vi "SIOSIfmDemo.vi"() -> ()   [LabVIEW 2009]
uses:
  SubVIs/Globals.vi
  <vilib>/Platform/TimedLoop/XDataNode/XDataNode.xnode
  <vilib>/Platform/TimedLoop/XDataNode/loadlvalarms.vi
  <vilib>/Platform/TimedLoop/XDataNode/timing_clust.ctl
  <vilib>/Platform/TimedLoop/XDataNode/nitl_modes.ctl
  <vilib>/Platform/TimedLoop/XDataNode/wakeup.ctl
  Instance           4 19Saved   SIOSIfmDemo .vi
  Instance           9 19Saved   SIOSIfmDemo .vi
  SIOS_IfmDLL/siosifm.dll
  <vilib>/Platform/TimedLoop/XDataNode/XDNodeRunTimeDep.lvlib
panel:
  in  "Registerkarte":T1(tab)
  out "Firmwareversion and date of compilation":string
  in  "COMNumber":i32=1 min=1 step=1
  in  "OpenCom":bool
  in  "Close":bool
  in  "CloseDevice":bool
  in  "OpenUSB":bool
  in  "Available Devices":i32(ring) items=["     1"]
  in  "SearchUSBDevices":bool
  in  "Init":bool
  in  "SetToZero":bool
  in  "StopMeasurement":bool
  in  "StartMeasurement":bool
  in  "GetMeasurement":bool
  in  "FireTrigger":bool
  in  "SetMeasurement":bool
  in  "StopSave":bool
  in  "SaveData":bool
  in  "Edge (on trigger input)":enum32{"Falling", "Rising"}(radio)
  in  "Start/Stop input":T2(radio)
  in  "Sample Clock":enum32{"Internal", "External"}(radio)
  in  "Edge (on clock input)":enum32{"Falling", "Rising"}(radio)
  in  "Hardware Trigger":bool
  in  "Edge (on event input)":enum32{"Falling", "Rising"}(radio)
  in  "Event input":enum32{"No function", "Single value"}(radio)
  in  "SampleCount":bool
  in  "Clock counter":bool
  in  "Circle":bool
  in  "SinCos":bool
  in  "Pattern":bool
  in  "Length":bool
  in  "OptionsFieldFilter":T3(radio)
  in  "Output word rate":dbl min=0.0 max=15000.0 step=10.0
  in  "Counter values":bool
  out "Channel 4":dbl
  out "Channel 3":dbl
  out "Channel 2":dbl
  out "Channel 1":dbl
  in  "Channel 4":bool
  in  "Channel 3":bool
  in  "Channel 2":bool
  in  "Channel 1":bool
  out "Estimated Outputwordrate":dbl format="%#_8f"
  in  "SetFilterBlockMode":bool
  in  "GetFilter":bool
  in  "FilterStage1NotchFreq":dbl caption="Channel 4" min=0.0
  in  "FilterStage1Ch4":dbl caption="Channel 4" min=0.0
  in  "FilterStage1Ch3":dbl caption="Channel 3" min=0.0
  in  "FilterStage1Ch2":dbl caption="Channel 2" min=0.0
  in  "FilterStage1Ch1":dbl caption="Channel 1" min=0.0
  in  "OptionFieldFilterStage1":T4(radio)
  in  "Filterstage2Val":u8 caption="2 to the power of"
  in  "9 times averaging active":bool
  in  "6 times averaging active":bool
  in  "5 times averaging active":bool
  in  "Filter stage 2":bool
  in  "Filter stage 1":bool
  in  "AVG1":u8 caption="2 to the power of"
  # "1. Initialze the DLL\n\n2. Select and open device (using USB-API or COM-port)"
  # "USB-API"
  # "COM-port"
  # "If all measurments are done, close device (Counterpart of \"OpenUSB\")"
  # "Close the library (Counterpart of \"Init\")"
  # "Signal processing options"
  # "Measurement values (length)"
  # "Measurement values selection"
  # "Filter stage 3"
  # "AVG 1"
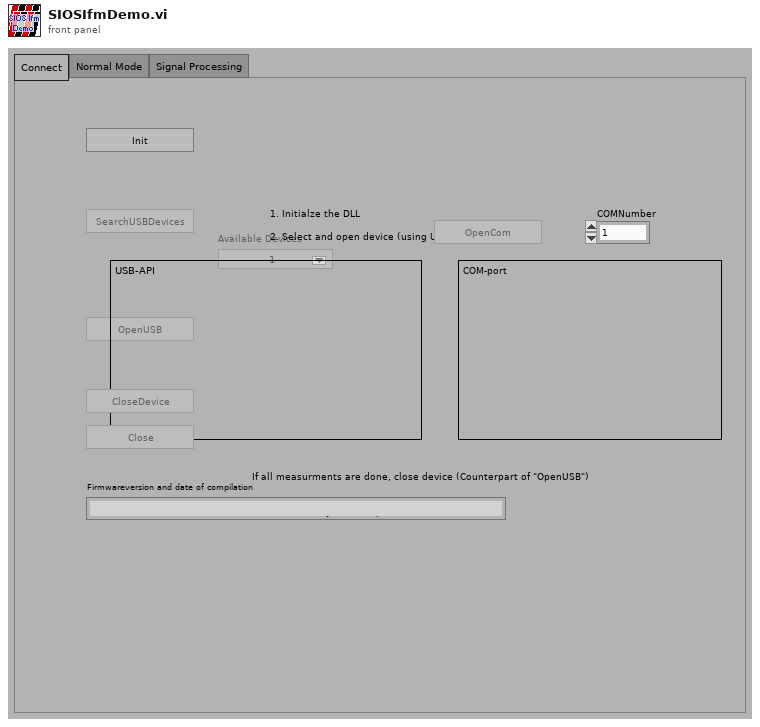
[diagram p1: front panel]
types:
  T1 = enum32{"Connect", "Normal Mode", "Signal Processing"}
  T2 = enum32{"No function", "Start trigger", "Start/Stop trigger", "Start/Stop processed"}
  T3 = enum32{"Filter off", "Filter default", "Filter user specified"}
  T4 = enum32{"FilterStage1Individual", "FilterStage1SupRefMirror", "FilterStage1NotchFilter"}
  T5 = enum8{"Enabled", "Disabled", "Disabled and Grayed Out"}
  T6 = typedef "XDNodeRunTimeDep.lvlib/timing_clust.ctl" = cluster{"Expected End [f-1]":u64, "Actual End [f-1]":u64, "Finished Late? [f-1]":bool, "Expected End [i-1]":u64, "Actual End [i-1]":u64, "Finished Late? [i-1]":bool, "Expected Start [i]":u64, "Actual Start [i]":u64, "Expected Start [f]":u64, "Actual Start [f]":u64, "Source Name":string, "Structure Name":string, "Period":i64, "Deadline":i64, "Offset":i64, "Start":i64, "Priority":i32, "Timeout":i32, "Mode":T7, "Wakeup Reason":T8, "Error":errorcluster, "Source Type":string, "Secondary Source Type":string, "Global End Time":u64, "Global Start Time":u64, "Frame Duration":u64, "Iteration Duration":u64, "Assigned CPU":i32, "I/O Scan Engine Mode":u32}
  T7 = typedef "XDNodeRunTimeDep.lvlib/nitl_modes.ctl" = enum32{"No Change", "Process missed periods, maintain original phase", "Discard missed periods, maintain original phase", "Process missed periods, ignore original phase", "Discard missed periods, ignore original phase"}
  T8 = typedef "XDNodeRunTimeDep.lvlib/wakeup.ctl" = enum32{"Normal", "Aborted", "Asynchronous wakeup", "Timing source error", "Timed loop error", "Timeout"}
  T9 = enum16{"open", "replace", "create", "open or create", "replace or create", "replace or create with confirmation"}
  T10 = cluster{"FilterOff":bool, "FilterAuto":bool, "FilterUserSpecified":bool, "FilterStage1":bool, "AVG1":i32, "FilterStage1CoeffCh1":dbl, "FilterStage1CoeffCh2":dbl, "FilterStage1CoeffCh3":dbl, "FilterStage1CoeffCh4":dbl, "FilterStage1NotchFreqCh1":dbl, "FilterStage1NotchFreqCh2":dbl, "FilterStage1NotchFreqCh3":dbl, "FilterStage1NotchFreqCh4":dbl, "FilterStage2":bool, "AVG2":i32, "5 times averaging active":bool, "6 times averaging active":bool, "9 times averaging active":bool}
  T11 = cluster{"TriggerModeOn":bool, "EventTriggerActivated":bool, "EdgeOnEventTrigger":bool, "ExternalClockActivated":bool, "EdgeOnExternalClock":bool, "TriggerStartActivated":bool, "TriggerStart/StopActivated":bool, "TriggerStart/StopProcessedActivated":bool, "EdgeOnTriggerInput":bool}
  T12 = cluster{"SendChannel1Data":bool, "SendChannel2Data":bool, "SendChannel3Data":bool, "SendChannel4Data":bool, "SendLengthValues":bool, "SendSinCosData":bool, "SendCircleData":bool, "SendTestPattern":bool, "SendClockCounterValue":bool, "SendSampleCounterValue":bool, "FilterSettings":enum32{"Auto filter", "Filter off", "Filter user specified"}, "OutputWordRate":i32}
  T13 = enum32{"Auto filter", "Filter off", "Filter user specified"}
  T14 = cluster{"Hardware Trigger":bool, "Start/Stop input":enum32{"No function", "Start trigger", "Start/Stop trigger", "Start/Stop processed"}, "Sample Clock":enum32{"Internal", "External"}, "Event input":enum32{"No function", "Single value"}, "Edge (on trigger input)":enum32{"Falling", "Rising"}, "Edge (on clock input)":enum32{"Falling", "Rising"}, "Edge (on event input)":enum32{"Falling", "Rising"}}
  T15 = cluster{"Value":bool, "Value":bool, "Value":bool, "Value":dbl, "Value":dbl, "Value":dbl, "Value":dbl, "Value":bool, "Value":dbl, "Value":bool, "Value":bool, "Value":bool, "Value":bool, "Value":u8, "Value":u8}
  T16 = cluster{"Channel 1":bool, "Channel 2":bool, "Channel 3":bool, "Channel 4":bool, "Length":bool, "SinCos":bool, "Circle":bool, "Pattern":bool, "Clock counter":bool, "SampleCount":bool, "OptionsFieldFilter":enum32{"Filter off", "Filter default", "Filter user specified"}, "Output word rate":dbl}
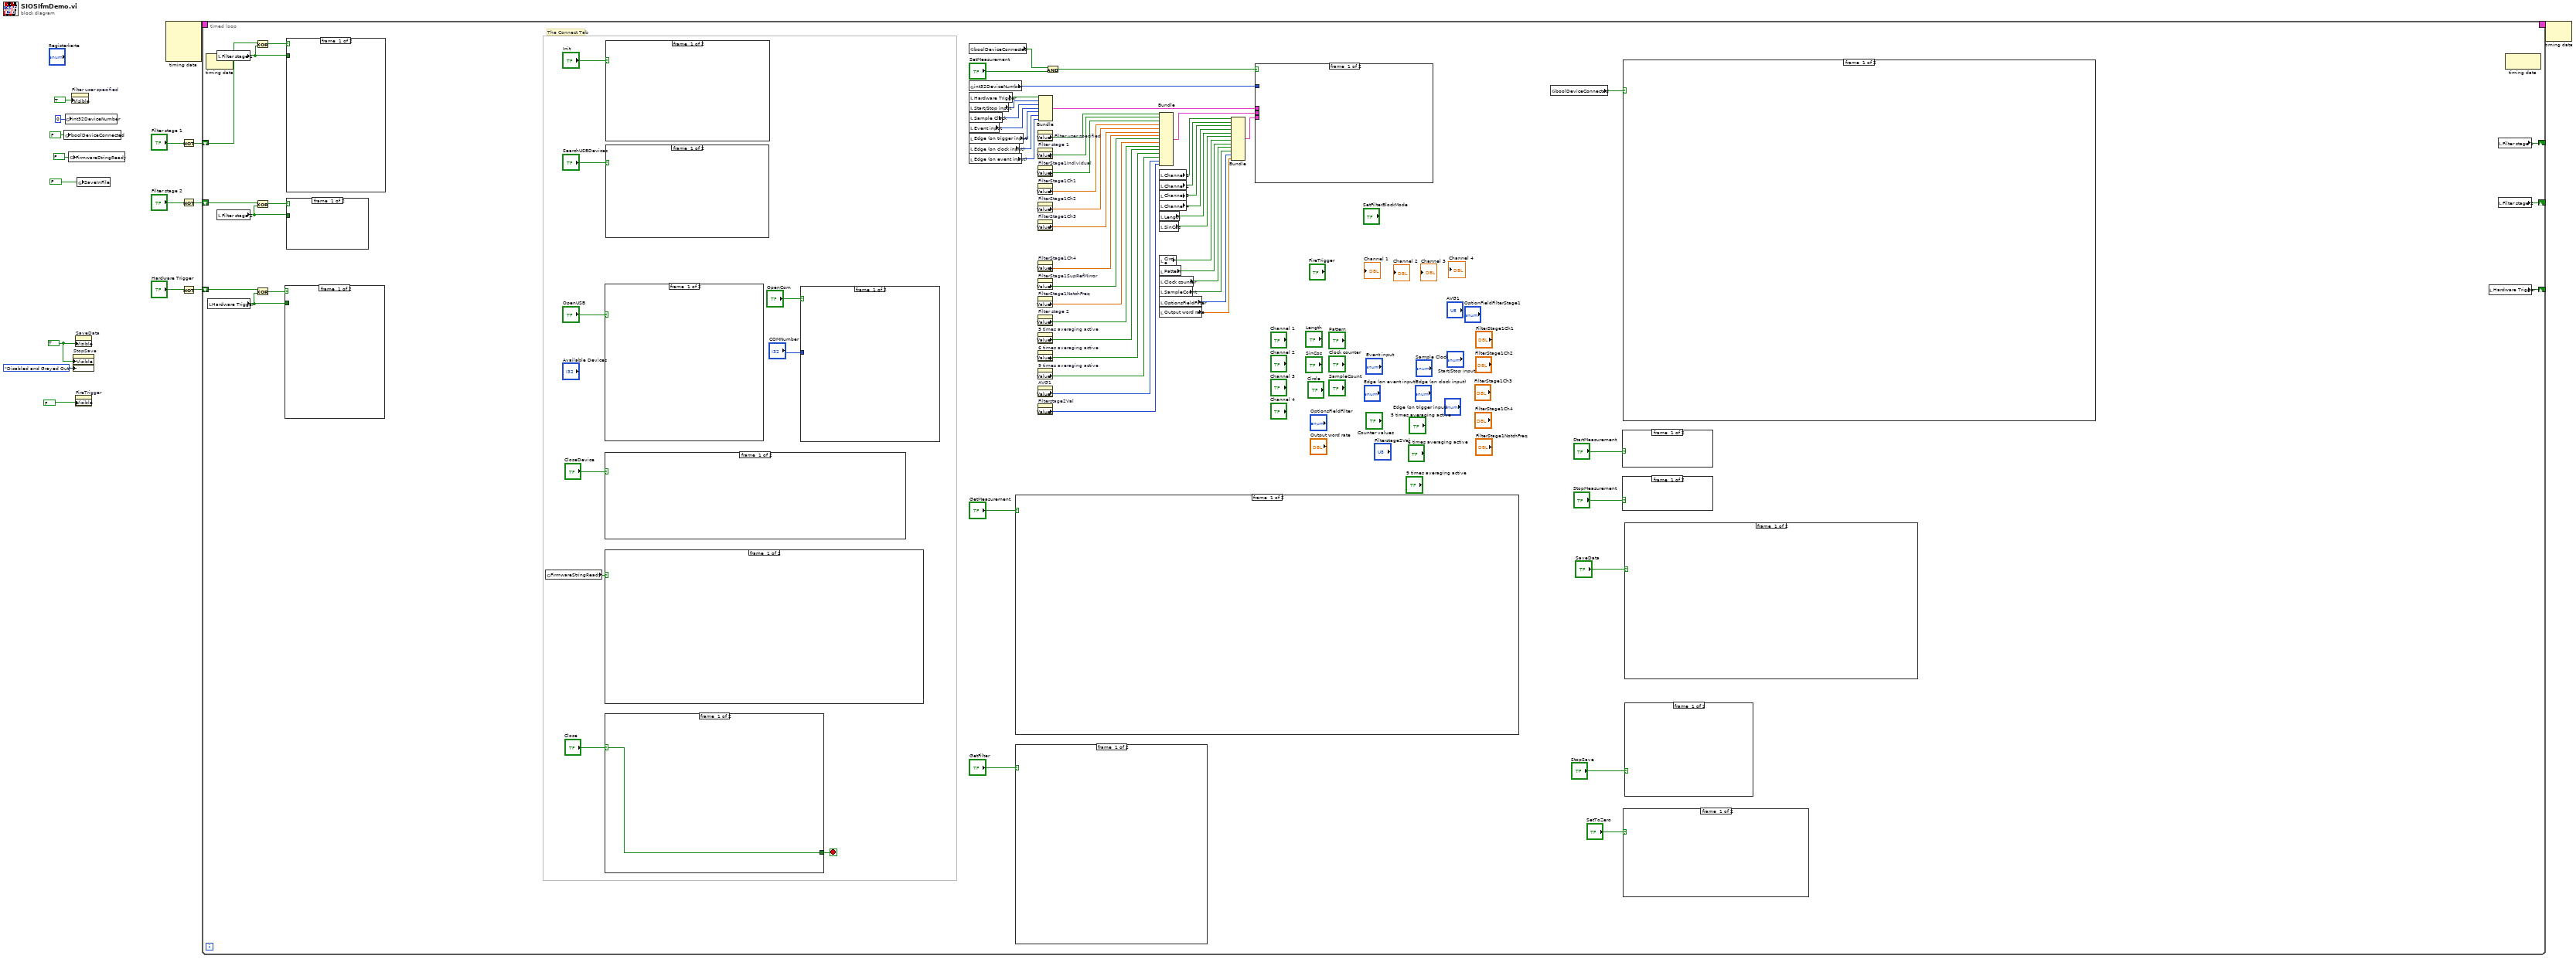
[diagram p0: block diagram]
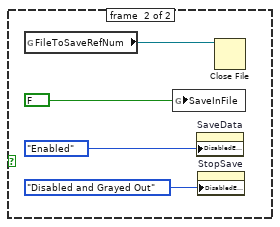
[diagram p2: hidden frame]
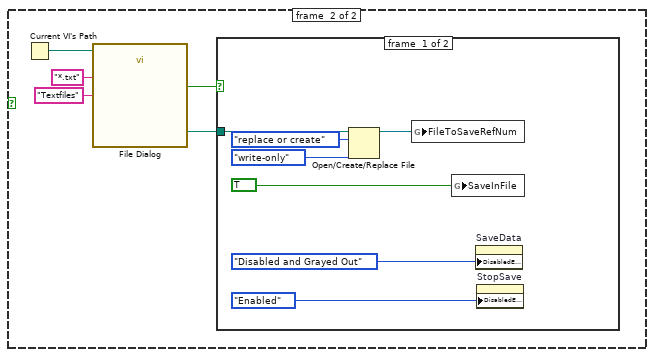
[diagram p3: hidden frame]
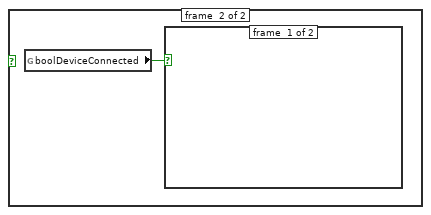
[diagram p5: hidden frame]
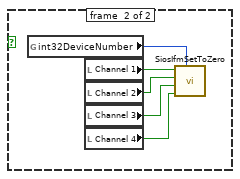
[diagram p6: hidden frame]
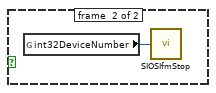
[diagram p7: hidden frame]
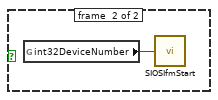
[diagram p8: hidden frame]
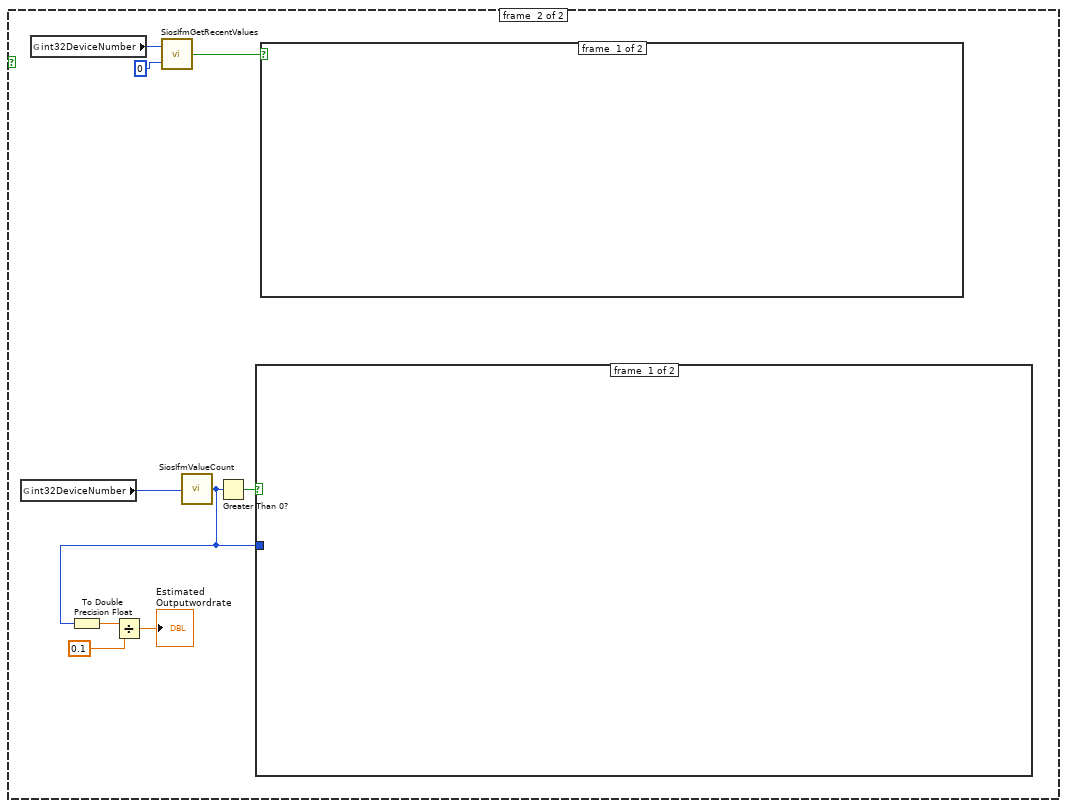
[diagram p9: hidden frame]
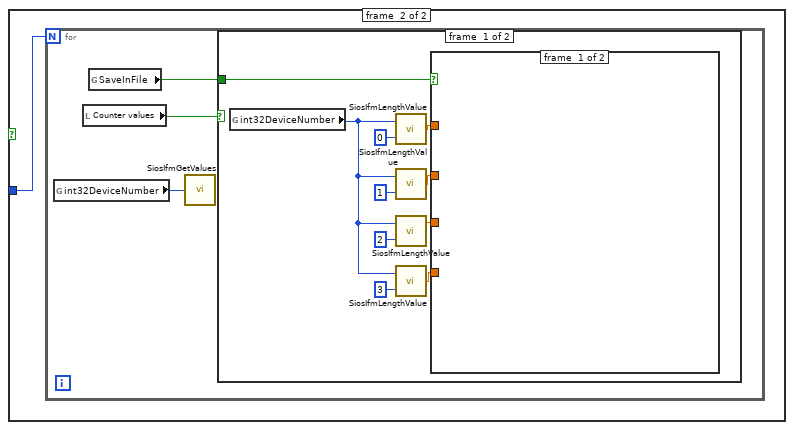
[diagram p10: hidden frame]
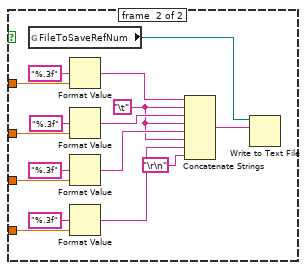
[diagram p11: hidden frame]
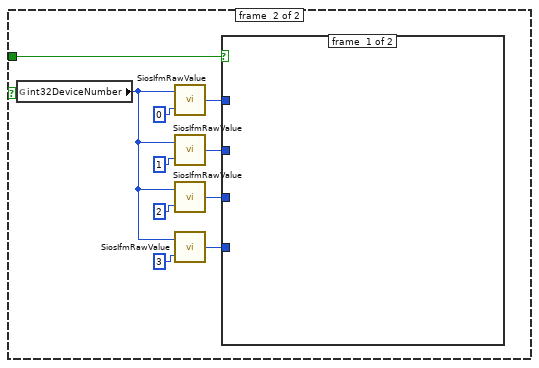
[diagram p12: hidden frame]
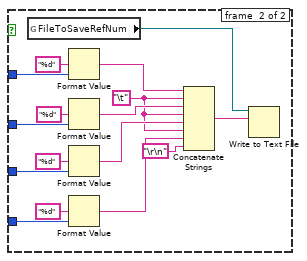
[diagram p13: hidden frame]
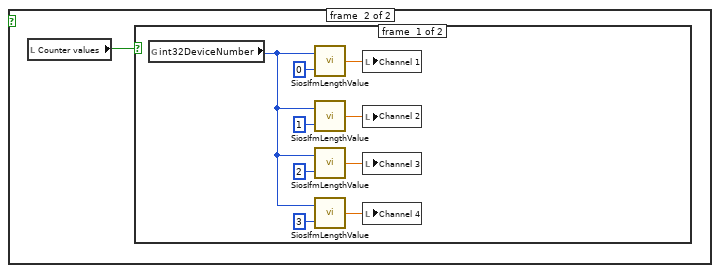
[diagram p14: hidden frame]
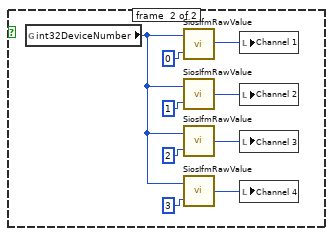
[diagram p15: hidden frame]
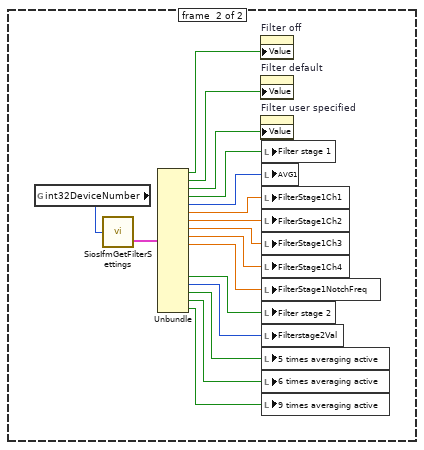
[diagram p16: hidden frame]
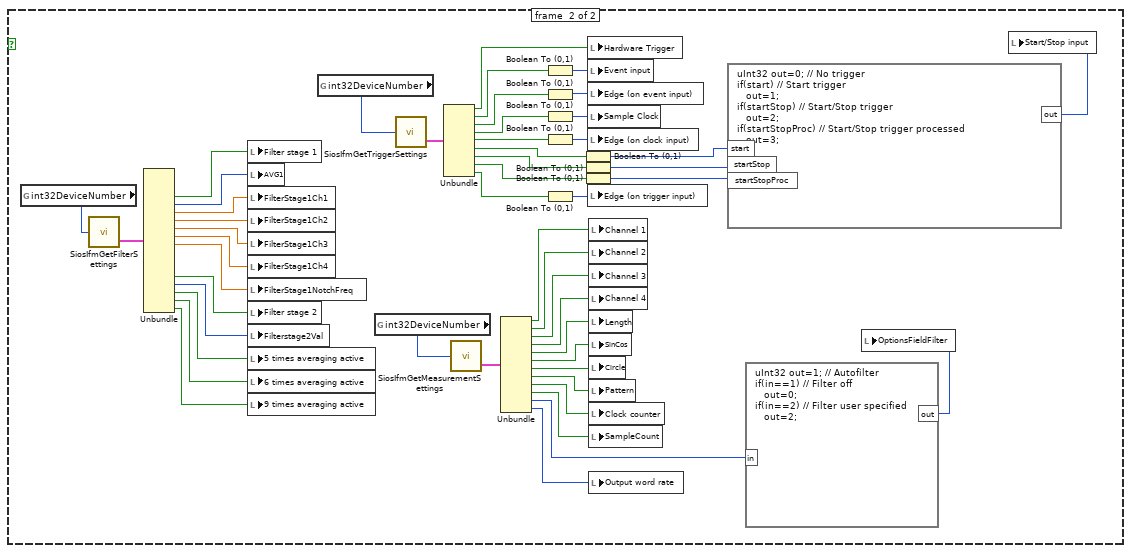
[diagram p17: hidden frame]
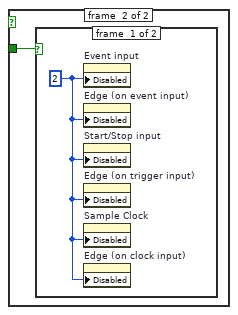
[diagram p18: hidden frame]
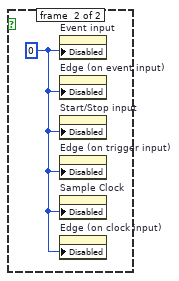
[diagram p19: hidden frame]
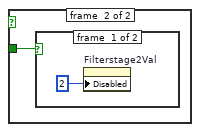
[diagram p20: hidden frame]
diagram:
  w4 = TRUE ("FirmwareStringReady")
  n1 = global write "Globals.vi" "boolDeviceConnected"(FALSE ("boolDeviceConnected")) -> ()
  n2 = global write "Globals.vi" "int32DeviceNumber"(0 ("int32DeviceNumber")) -> ()
  n3 = global write "Globals.vi" "FirmwareStringReady"(FALSE ("FirmwareStringReady")) -> ()
  n4 = property on="Filter user specified" class="Boolesch (strikt)"("Visible"=TRUE ("Sichtbar")) -> ()  [unwired: 2 in, 2 out]
  n5 = property on="StopSave" class="Bool"("Visible"=w4, "DisabledEnum"=T5."Disabled and Grayed Out" ("Disabled")) -> ()  [unwired: 2 in, 2 out]
  n6 = property on="SaveData" class="Bool"("Visible"=w4) -> ()  [unwired: 2 in, 2 out]
  n7 = property on="FireTrigger" class="Bool"("Visible"=FALSE ("FirmwareStringReady")) -> ()  [unwired: 2 in, 2 out]
  n8 = global write "Globals.vi" "SaveInFile"(FALSE ("FirmwareStringReady")) -> ()
  n9 = node-c288() -> (w6:T6)  [unwired: 4 in]
  n10 = Not(x="Filter stage 1") -> (.not. x?=w12:bool)
  n11 = Not(x="Filter stage 2") -> (.not. x?=w10:bool)
  n12 = Not(x="Hardware Trigger") -> (.not. x?=w9:bool)
  n13 = timed-loop {
    shift-right: [w55] -> _
    shift-left: w12 -> [w51]
    shift-right: [w54] -> _
    shift-left: w10 -> [w50]
    shift-right: [w52] -> _
    shift-left: w9 -> [w49]
    timing: w6 -> [_]
    timing-out: [_] -> w5
    stop <- w84 stop-if-true
    # "The Connect Tab"
    n14 = node-c288() -> ()  [unwired: 1 in, 1 out]
    n15 = local read "Hardware Trigger"() -> (w43:bool)
    n16 = local read "Filter stage 1"() -> (w47:bool)
    n17 = local read "Filter stage 2"() -> (w45:bool)
    n18 = Exclusive Or(1:w47, 2:w51) -> (0:w48:bool)
    n19 = Exclusive Or(1:w45, 2:w50) -> (0:w46:bool)
    n20 = Exclusive Or(1:w43, 2:w49) -> (0:w44:bool)
    n21 = case shown="True" w44 {
      tunnel: w43 -> [_ w263]
      frame #0 {
      }
      frame #1 {
        n22 = case shown="False" w263 {
          frame #0 {
            w264 = u8 2 ("Nicht aktiv")
            n23 = property on="Event input" class="OptionsfelderElement (strikt)"("Disabled"=w264) -> ()  [unwired: 2 in, 2 out]
            n24 = property on="Edge (on event input)" class="OptionsfelderElement (strikt)"("Disabled"=w264) -> ()  [unwired: 2 in, 2 out]
            n25 = property on="Start/Stop input" class="OptionsfelderElement (strikt)"("Disabled"=w264) -> ()  [unwired: 2 in, 2 out]
            n26 = property on="Edge (on trigger input)" class="OptionsfelderElement (strikt)"("Disabled"=w264) -> ()  [unwired: 2 in, 2 out]
            n27 = property on="Sample Clock" class="OptionsfelderElement (strikt)"("Disabled"=w264) -> ()  [unwired: 2 in, 2 out]
            n28 = property on="Edge (on clock input)" class="OptionsfelderElement (strikt)"("Disabled"=w264) -> ()  [unwired: 2 in, 2 out]
          }
          frame #1 {
            w265 = u8 0 ("Nicht aktiv")
            n29 = property on="Event input" class="OptionsfelderElement (strikt)"("Disabled"=w265) -> ()  [unwired: 2 in, 2 out]
            n30 = property on="Edge (on event input)" class="OptionsfelderElement (strikt)"("Disabled"=w265) -> ()  [unwired: 2 in, 2 out]
            n31 = property on="Start/Stop input" class="OptionsfelderElement (strikt)"("Disabled"=w265) -> ()  [unwired: 2 in, 2 out]
            n32 = property on="Edge (on trigger input)" class="OptionsfelderElement (strikt)"("Disabled"=w265) -> ()  [unwired: 2 in, 2 out]
            n33 = property on="Sample Clock" class="OptionsfelderElement (strikt)"("Disabled"=w265) -> ()  [unwired: 2 in, 2 out]
            n34 = property on="Edge (on clock input)" class="OptionsfelderElement (strikt)"("Disabled"=w265) -> ()  [unwired: 2 in, 2 out]
          }
        }
      }
    }
    n35 = case shown="True" w48 {
      tunnel: w47 -> [_ w269]
      frame #0 {
      }
      frame #1 {
        n36 = case shown="True" w269 {
          frame #0 {
            w270 = u8 2 ("Nicht aktiv")
            n37 = property on="AVG1" class="Digital (strikt)"("Disabled"=w270) -> ()  [unwired: 2 in, 2 out]
            n38 = property on="OptionFieldFilterStage1" class="OptionsfelderElement (strikt)"("Disabled"=w270) -> ()  [unwired: 2 in, 2 out]
            n39 = property on="FilterStage1Ch1" class="Digital (strikt)"("Disabled"=w270) -> ()  [unwired: 2 in, 2 out]
            n40 = property on="FilterStage1Ch2" class="DigitalWert (strikt)"("Disabled"=w270) -> ()  [unwired: 2 in, 2 out]
            n41 = property on="FilterStage1Ch3" class="DigitalWert (strikt)"("Disabled"=w270) -> ()  [unwired: 2 in, 2 out]
            n42 = property on="FilterStage1Ch4" class="DigitalWert (strikt)"("Disabled"=w270) -> ()  [unwired: 2 in, 2 out]
            n43 = property on="FilterStage1NotchFreq" class="Digital (strikt)"("Disabled"=w270) -> ()  [unwired: 2 in, 2 out]
          }
          frame #1 {
            w271 = u8 0 ("Nicht aktiv")
            n44 = property on="AVG1" class="Digital (strikt)"("Disabled"=w271) -> ()  [unwired: 2 in, 2 out]
            n45 = property on="OptionFieldFilterStage1" class="OptionsfelderElement (strikt)"("Disabled"=w271) -> ()  [unwired: 2 in, 2 out]
            n46 = property on="FilterStage1Ch1" class="Digital (strikt)"("Disabled"=w271) -> ()  [unwired: 2 in, 2 out]
            n47 = property on="FilterStage1Ch2" class="DigitalWert (strikt)"("Disabled"=w271) -> ()  [unwired: 2 in, 2 out]
            n48 = property on="FilterStage1Ch3" class="DigitalWert (strikt)"("Disabled"=w271) -> ()  [unwired: 2 in, 2 out]
            n49 = property on="FilterStage1Ch4" class="DigitalWert (strikt)"("Disabled"=w271) -> ()  [unwired: 2 in, 2 out]
            n50 = property on="FilterStage1NotchFreq" class="Digital (strikt)"("Disabled"=w271) -> ()  [unwired: 2 in, 2 out]
          }
        }
      }
    }
    n51 = case shown="True" w46 {
      tunnel: w45 -> [_ w266]
      frame #0 {
      }
      frame #1 {
        n52 = case shown="False" w266 {
          frame #0 {
            n53 = property on="Filterstage2Val" class="Digital (strikt)"("Disabled"=u8 2 ("Nicht aktiv")) -> ()  [unwired: 2 in, 2 out]
          }
          frame #1 {
            n54 = property on="Filterstage2Val" class="Digital (strikt)"("Disabled"=u8 0 ("Nicht aktiv")) -> ()  [unwired: 2 in, 2 out]
          }
        }
      }
    }
    n55 = global read "Globals.vi" "FirmwareStringReady"() -> (w78:bool)
    n56 = case shown="True" "OpenUSB" {
      frame #0 {
      }
      frame #1 {
        n57 = property on="Available Devices" class="Ring (strikt)"() -> ("Value"=w295:i32)  [unwired: 2 in, 2 out]
        n58 = call "SiosIfmOpenUSB.vi"("uniqueId"=w295) -> ("IfmOpenUSB"=w296:i32)
        n59 = Greater Or Equal To 0?(x=w296) -> (x >= 0?=w297:bool)
        n60 = case shown="True" w297 {
          tunnel: w296 -> [_ w299]
          frame #0 {
          }
          frame #1 {
            w301 = u8 2 ("Nicht aktiv")
            n61 = global write "Globals.vi" "int32DeviceNumber"(w299) -> ()
            n62 = global write "Globals.vi" "boolDeviceConnected"(TRUE ("boolDeviceConnected")) -> ()
            n63 = global write "Globals.vi" "FirmwareStringReady"(TRUE ("FirmwareStringReady")) -> ()
            n64 = property on="CloseDevice" class="Boolesch"("Disabled"=u8 0 ("Nicht aktiv")) -> ()  [unwired: 2 in, 2 out]
            n65 = property on="OpenUSB" class="Boolesch"("Disabled"=w301) -> ()  [unwired: 2 in, 2 out]
            n66 = property on="OpenCom" class="Boolesch"("Disabled"=w301) -> ()  [unwired: 2 in, 2 out]
          }
        }
      }
    }
    n67 = case shown="True" "CloseDevice" {
      frame #0 {
      }
      frame #1 {
        n68 = flat-sequence {
          frame #0 {
            n69 = global read "Globals.vi" "int32DeviceNumber"() -> (w292:i32)
            n70 = call "SiosIfmCloseDevice.vi"("DeviceNumber"=w292) -> ()
          }
          frame #1 {
            w294 = u8 0 ("Nicht aktiv")
            n71 = property on="CloseDevice" class="Boolesch"("Disabled"=u8 2 ("Nicht aktiv")) -> ()  [unwired: 2 in, 2 out]
            n72 = property on="OpenUSB" class="Boolesch"("Disabled"=w294) -> ()  [unwired: 2 in, 2 out]
            n73 = property on="OpenCom" class="Boolesch"("Disabled"=w294) -> ()  [unwired: 2 in, 2 out]
          }
        }
        n74 = global write "Globals.vi" "boolDeviceConnected"(FALSE ("boolDeviceConnected")) -> ()
      }
    }
    n75 = case shown="True" w78 {
      frame #0 {
      }
      frame #1 {
        n76 = flat-sequence {
          frame #0 {
            n77 = while {
              i -> [w285]
              stop <- w283 continue-if-true
              # "Wait until\ndevice info\nis available\nor timeout \nafter \n5 seconds."
              n78 = global read "Globals.vi" "int32DeviceNumber"() -> (w278:i32)
              n79 = Greater Or Equal?(x=50, y=w285) -> (x >= y?=w281:bool)
              n80 = call "Verzögerung"("Delay Time (s)"=0.1) -> ()  [unwired: 10 in, 1 out]
              n81 = dll-call lib="D:/Support/Labview/RE-10/SIOS_IfmDLL/siosifm.dll" fn="IfmDeviceInfo"("deviceNumber"=w278, "requestedInfo"=8) -> (w279:i32)  [unwired: 5 in, 2 out]
              n82 = Not Equal?(x=1, y=w279) -> (x != y?=w282:bool)
              n83 = And(x=w282, y=w281) -> (x .and. y?=w283:bool)
            }
          }
          frame #1 {
            n84 = global read "Globals.vi" "int32DeviceNumber"() -> (w288:i32)
            n85 = global write "Globals.vi" "FirmwareStringReady"(FALSE ("FirmwareStringReady")) -> ()
            n86 = call "SiosIfmIGetFirmwareVersion.vi"("devNumber"=w288) -> ("Ausgabe-Parameter"=→"Firmwareversion and date of compilation":string)
          }
        }
      }
    }
    n87 = case shown="True" "Close" {
      selector: "Close" -> [w317 w320]
      tunnel: [w317 w318] -> w84
      frame #0 {
      }
      frame #1 {
        n88 = flat-sequence {
          tunnel: w320 -> [w321]
          tunnel: [w321] -> w319
          tunnel: [w324] -> w318
          tunnel: w319 -> [w324]
          frame #0 {
            n89 = call "SIOSIfmClose.vi"() -> ()  [unwired: 1 in]
          }
          frame #1 {
            w323 = u8 2 ("Nicht aktiv")
            n90 = property on="Init" class="Boolesch"("Disabled"=u8 0 ("Nicht aktiv")) -> ()  [unwired: 2 in, 2 out]
            n91 = property on="SearchUSBDevices" class="Boolesch"("Disabled"=w323) -> ()  [unwired: 2 in, 2 out]
            n92 = property on="OpenUSB" class="Boolesch"("Disabled"=w323) -> ()  [unwired: 2 in, 2 out]
            n93 = property on="Available Devices" class="Ring (strikt)"("Disabled"=w323) -> ()  [unwired: 2 in, 2 out]
            n94 = global write "Globals.vi" "boolDeviceConnected"(FALSE ("boolDeviceConnected")) -> ()
            n95 = property on="CloseDevice" class="Boolesch"("Disabled"=w323) -> ()  [unwired: 2 in, 2 out]
            n96 = property on="Close" class="Boolesch"("Disabled"=w323) -> ()  [unwired: 2 in, 2 out]
            n97 = property on="OpenCom" class="Boolesch"("Disabled"=w323) -> ()  [unwired: 2 in, 2 out]
          }
        }
      }
    }
    n98 = case shown="True" "Init" {
      frame #0 {
      }
      frame #1 {
        n99 = call "SiosIfmInit.vi"() -> ("IfmInit"=w326:i32)
        n100 = Equal To 0?(x=w326) -> (x = 0?=w327:bool)
        n101 = case shown="True" w327 {
          frame #0 {
          }
          frame #1 {
            w328 = u8 0 ("Nicht aktiv")
            n102 = property on="Init" class="Boolesch"("Disabled"=u8 2 ("Nicht aktiv")) -> ()  [unwired: 2 in, 2 out]
            n103 = property on="SearchUSBDevices" class="Boolesch"("Disabled"=w328) -> ()  [unwired: 2 in, 2 out]
            n104 = property on="Close" class="Boolesch"("Disabled"=w328) -> ()  [unwired: 2 in, 2 out]
            n105 = property on="OpenCom" class="Boolesch"("Disabled"=w328) -> ()  [unwired: 2 in, 2 out]
          }
        }
      }
    }
    n106 = case shown="True" "SearchUSBDevices" {
      frame #0 {
      }
      frame #1 {
        n107 = call "SiosIfmSearchUSBDevices.vi"() -> ("Array"=w312:cluster{string, i16}[], "Number of SIOS USB Devices"=w313:i32)
        n108 = Greater Than 0?(x=w313) -> (x > 0?=w311:bool)
        n109 = case shown="True" w311 {
          tunnel: w312 -> [_ w314]
          frame #0 {
          }
          frame #1 {
            n110 = property on="Available Devices" class="Ring (strikt)"("Strings And Values []"=w314) -> ()  [unwired: 2 in, 2 out]
            n111 = property on="OpenUSB" class="Boolesch"("Disabled"=u8 0 ("Nicht aktiv")) -> ()  [unwired: 2 in, 2 out]
            n112 = property on="Available Devices" class="Ring (strikt)"("Disabled"=u8 0 ("Nicht aktiv")) -> ()  [unwired: 2 in, 2 out]
          }
        }
      }
    }
    n113 = case shown="True" "OpenCom" {
      tunnel: "COMNumber" -> [_ w305]
      frame #0 {
      }
      frame #1 {
        n114 = dll-call lib="D:/Support/Labview/RE-10/SIOS_IfmDLL/siosifm.dll" fn="IfmOpenCOM"("ComNumber"=w305) -> (w303:i32)  [unwired: 4 in, 2 out]
        n115 = Greater Or Equal To 0?(x=w303) -> (x >= 0?=w304:bool)
        n116 = case shown="True" w304 {
          tunnel: w303 -> [_ w307]
          frame #0 {
          }
          frame #1 {
            w309 = u8 2 ("Nicht aktiv")
            n117 = global write "Globals.vi" "int32DeviceNumber"(w307) -> ()
            n118 = global write "Globals.vi" "boolDeviceConnected"(TRUE ("boolDeviceConnected")) -> ()
            n119 = global write "Globals.vi" "FirmwareStringReady"(TRUE ("FirmwareStringReady")) -> ()
            n120 = property on="CloseDevice" class="Boolesch"("Disabled"=u8 0 ("Nicht aktiv")) -> ()  [unwired: 2 in, 2 out]
            n121 = property on="OpenUSB" class="Boolesch"("Disabled"=w309) -> ()  [unwired: 2 in, 2 out]
            n122 = property on="OpenCom" class="Boolesch"("Disabled"=w309) -> ()  [unwired: 2 in, 2 out]
          }
        }
      }
    }
    n123 = global read "Globals.vi" "boolDeviceConnected"() -> (w58:bool)
    n124 = global read "Globals.vi" "int32DeviceNumber"() -> (w76:i32)
    n125 = local read "Hardware Trigger"() -> (w53:bool)
    n126 = local read "Start/Stop input"() -> (w28:T2)
    n127 = local read "Sample Clock"() -> (w27:enum32{"Internal", "External"})
    n128 = local read "Event input"() -> (w26:enum32{"No function", "Single value"})
    n129 = local read "Edge (on trigger input)"() -> (w25:enum32{"Falling", "Rising"})
    n130 = local read "Edge (on clock input)"() -> (w24:enum32{"Falling", "Rising"})
    n131 = local read "Edge (on event input)"() -> (w23:enum32{"Falling", "Rising"})
    n132 = case shown="True" "GetMeasurement" {
      frame #0 {
      }
      frame #1 {
        n133 = global read "Globals.vi" "int32DeviceNumber"() -> (w262:i32)
        n134 = call "SiosIfmGetFilterSettings.vi"("devNumber"=w262) -> ("FilterSettings"=w261:T10)  [unwired: 1 out]
        n135 = Unbundle(w261) -> ("FilterStage1"=w260:bool, "AVG1"=w259:i32, "FilterStage1CoeffCh1"=w258:dbl, "FilterStage1CoeffCh2"=w257:dbl, "FilterStage1CoeffCh3"=w256:dbl, "FilterStage1CoeffCh4"=w255:dbl, "FilterStage1NotchFreqCh1"=w254:dbl, "FilterStage2"=w253:bool, "AVG2"=w252:i32, "5 times averaging active"=w251:bool, "6 times averaging active"=w250:bool, "9 times averaging active"=w249:bool)  [unwired: 6 out]
        n136 = local write "Filter stage 1"(w260) -> ()
        n137 = local write "AVG1"(w259) -> ()
        n138 = local write "FilterStage1Ch1"(w258) -> ()
        n139 = local write "FilterStage1Ch2"(w257) -> ()
        n140 = local write "FilterStage1Ch3"(w256) -> ()
        n141 = local write "FilterStage1Ch4"(w255) -> ()
        n142 = local write "FilterStage1NotchFreq"(w254) -> ()
        n143 = local write "Filter stage 2"(w253) -> ()
        n144 = local write "Filterstage2Val"(w252) -> ()
        n145 = local write "5 times averaging active"(w251) -> ()
        n146 = local write "6 times averaging active"(w250) -> ()
        n147 = local write "9 times averaging active"(w249) -> ()
        n148 = global read "Globals.vi" "int32DeviceNumber"() -> (w236:i32)
        n149 = global read "Globals.vi" "int32DeviceNumber"() -> (w216:i32)
        n150 = call "SiosIfmGetTriggerSettings.vi"("devNumber"=w236) -> ("TriggerSettings"=w237:T11)  [unwired: 1 out]
        n151 = Unbundle(w237) -> ("TriggerModeOn"=w238:bool, "EventTriggerActivated"=w239:bool, "EdgeOnEventTrigger"=w243:bool, "ExternalClockActivated"=w244:bool, "EdgeOnExternalClock"=w246:bool, "TriggerStartActivated"=w235:bool, "TriggerStart/StopActivated"=w234:bool, "TriggerStart/StopProcessedActivated"=w229:bool, "EdgeOnTriggerInput"=w248:bool)
        n152 = call "SiosIfmGetMeasurementSettings.vi"("devNumber"=w216) -> ("MeasurementSettings"=w217:T12)  [unwired: 1 out]
        n153 = Unbundle(w217) -> ("SendChannel1Data"=w218:bool, "SendChannel2Data"=w219:bool, "SendChannel3Data"=w220:bool, "SendChannel4Data"=w221:bool, "SendLengthValues"=w222:bool, "SendSinCosData"=w223:bool, "SendCircleData"=w228:bool, "SendTestPattern"=w227:bool, "SendClockCounterValue"=w226:bool, "SendSampleCounterValue"=w225:bool, "FilterSettings"=w215:T13, "OutputWordRate"=w224:i32)
        n154 = Boolean To (0,1)(Boolean=w239) -> (0, 1=w240:i16)
        n155 = Boolean To (0,1)(Boolean=w243) -> (0, 1=w241:i16)
        n156 = Boolean To (0,1)(Boolean=w244) -> (0, 1=w242:i16)
        n157 = Boolean To (0,1)(Boolean=w246) -> (0, 1=w245:i16)
        n158 = Boolean To (0,1)(Boolean=w248) -> (0, 1=w247:i16)
        n159 = Boolean To (0,1)(Boolean=w235) -> (0, 1=w233:i16)
        n160 = Boolean To (0,1)(Boolean=w234) -> (0, 1=w232:i16)
        n161 = Boolean To (0,1)(Boolean=w229) -> (0, 1=w231:i16)
        n162 = local write "Hardware Trigger"(w238) -> ()
        n163 = local write "Event input"(w240) -> ()
        n164 = local write "Edge (on event input)"(w241) -> ()
        n165 = local write "Sample Clock"(w242) -> ()
        n166 = local write "Edge (on clock input)"(w245) -> ()
        n167 = local write "Edge (on trigger input)"(w247) -> ()
        n168 = local write "Channel 1"(w218) -> ()
        n169 = local write "Channel 2"(w219) -> ()
        n170 = local write "Channel 3"(w220) -> ()
        n171 = local write "Channel 4"(w221) -> ()
        n172 = local write "Length"(w222) -> ()
        n173 = local write "SinCos"(w223) -> ()
        n174 = local write "Circle"(w228) -> ()
        n175 = local write "Pattern"(w227) -> ()
        n176 = local write "Clock counter"(w226) -> ()
        n177 = local write "SampleCount"(w225) -> ()
        n178 = local write "Output word rate"(w224) -> ()
        n179 = formula code="uInt32 out=0; // No trigger\nif(start) // Start trigger\n   out=1;\nif(startStop) // Start/Stop trigger\n   out=2;\nif(startStopProc) // Start/Stop trigger processed\n   out=3;"("start"=w233, "startStop"=w232, "startStopProc"=w231) -> ("out"=w230:u32)
        n180 = formula code="uInt32 out=1; // Autofilter\nif(in==1) // Filter off\n   out=0;\nif(in==2) // Filter user specified\n   out=2;"("in"=w215) -> ("out"=w214:u32)
        n181 = local write "OptionsFieldFilter"(w214) -> ()
        n182 = local write "Start/Stop input"(w230) -> ()
      }
    }
    n183 = case shown="True" "GetFilter" {
      frame #0 {
      }
      frame #1 {
        n184 = global read "Globals.vi" "int32DeviceNumber"() -> (w197:i32)
        n185 = call "SiosIfmGetFilterSettings.vi"("devNumber"=w197) -> ("FilterSettings"=w198:T10)  [unwired: 1 out]
        n186 = Unbundle(w198) -> ("FilterOff"=w199:bool, "FilterAuto"=w200:bool, "FilterUserSpecified"=w201:bool, "FilterStage1"=w202:bool, "AVG1"=w203:i32, "FilterStage1CoeffCh1"=w204:dbl, "FilterStage1CoeffCh2"=w205:dbl, "FilterStage1CoeffCh3"=w206:dbl, "FilterStage1CoeffCh4"=w207:dbl, "FilterStage1NotchFreqCh1"=w208:dbl, "FilterStage2"=w209:bool, "AVG2"=w210:i32, "5 times averaging active"=w211:bool, "6 times averaging active"=w212:bool, "9 times averaging active"=w213:bool)  [unwired: 3 out]
        n187 = property on="Filter off" class="Boolesch (strikt)"("Value"=w199) -> ()  [unwired: 2 in, 2 out]
        n188 = property on="Filter default" class="Boolesch (strikt)"("Value"=w200) -> ()  [unwired: 2 in, 2 out]
        n189 = property on="Filter user specified" class="Boolesch (strikt)"("Value"=w201) -> ()  [unwired: 2 in, 2 out]
        n190 = local write "Filter stage 1"(w202) -> ()
        n191 = local write "AVG1"(w203) -> ()
        n192 = local write "FilterStage1Ch1"(w204) -> ()
        n193 = local write "FilterStage1Ch2"(w205) -> ()
        n194 = local write "FilterStage1Ch3"(w206) -> ()
        n195 = local write "FilterStage1Ch4"(w207) -> ()
        n196 = local write "FilterStage1NotchFreq"(w208) -> ()
        n197 = local write "Filter stage 2"(w209) -> ()
        n198 = local write "Filterstage2Val"(w210) -> ()
        n199 = local write "5 times averaging active"(w211) -> ()
        n200 = local write "6 times averaging active"(w212) -> ()
        n201 = local write "9 times averaging active"(w213) -> ()
      }
    }
    n202 = property on="Filter user specified" class="Boolesch (strikt)"() -> ("Value"=w75:bool)  [unwired: 2 in, 2 out]
    n203 = property on="Filter stage 1" class="Boolesch (strikt)"() -> ("Value"=w74:bool)  [unwired: 2 in, 2 out]
    n204 = property on="FilterStage1Individual" class="Boolesch (strikt)"() -> ("Value"=w73:bool)  [unwired: 2 in, 2 out]
    n205 = property on="FilterStage1Ch1" class="Digital (strikt)"() -> ("Value"=w72:dbl)  [unwired: 2 in, 2 out]
    n206 = property on="FilterStage1Ch2" class="DigitalWert (strikt)"() -> ("Value"=w71:dbl)  [unwired: 2 in, 2 out]
    n207 = property on="FilterStage1Ch3" class="DigitalWert (strikt)"() -> ("Value"=w70:dbl)  [unwired: 2 in, 2 out]
    n208 = property on="FilterStage1Ch4" class="DigitalWert (strikt)"() -> ("Value"=w69:dbl)  [unwired: 2 in, 2 out]
    n209 = property on="FilterStage1SupRefMirror" class="Boolesch (strikt)"() -> ("Value"=w68:bool)  [unwired: 2 in, 2 out]
    n210 = property on="FilterStage1NotchFreq" class="Digital (strikt)"() -> ("Value"=w67:dbl)  [unwired: 2 in, 2 out]
    n211 = property on="Filter stage 2" class="Boolesch (strikt)"() -> ("Value"=w66:bool)  [unwired: 2 in, 2 out]
    n212 = property on="5 times averaging active" class="Boolesch (strikt)"() -> ("Value"=w65:bool)  [unwired: 2 in, 2 out]
    n213 = property on="6 times averaging active" class="Boolesch (strikt)"() -> ("Value"=w64:bool)  [unwired: 2 in, 2 out]
    n214 = property on="9 times averaging active" class="Boolesch (strikt)"() -> ("Value"=w63:bool)  [unwired: 2 in, 2 out]
    n215 = property on="AVG1" class="Digital (strikt)"() -> ("Value"=w62:u8)  [unwired: 2 in, 2 out]
    n216 = property on="Filterstage2Val" class="Digital (strikt)"() -> ("Value"=w61:u8)  [unwired: 2 in, 2 out]
    n217 = Bundle("Hardware Trigger"=w53, "Start/Stop input"=w28, "Sample Clock"=w27, "Event input"=w26, "Edge (on trigger input)"=w25, "Edge (on clock input)"=w24, "Edge (on event input)"=w23) -> (w77:T14)  [unwired: 1 in]
    n218 = And(x=w58, y="SetMeasurement") -> (x .and. y?=w56:bool)
    n219 = Bundle("Value"=w75, "Value"=w74, "Value"=w73, "Value"=w72, "Value"=w71, "Value"=w70, "Value"=w69, "Value"=w68, "Value"=w67, "Value"=w66, "Value"=w65, "Value"=w64, "Value"=w63, "Value"=w62, "Value"=w61) -> (w60:T15)  [unwired: 1 in]
    n220 = local read "Channel 1"() -> (w40:bool)
    n221 = local read "Channel 2"() -> (w39:bool)
    n222 = local read "Channel 3"() -> (w38:bool)
    n223 = local read "Channel 4"() -> (w37:bool)
    n224 = local read "Length"() -> (w36:bool)
    n225 = local read "SinCos"() -> (w35:bool)
    n226 = local read "Circle"() -> (w34:bool)
    n227 = local read "Pattern"() -> (w33:bool)
    n228 = local read "Clock counter"() -> (w32:bool)
    n229 = local read "SampleCount"() -> (w31:bool)
    n230 = local read "OptionsFieldFilter"() -> (w30:T3)
    n231 = local read "Output word rate"() -> (w29:dbl)
    n232 = Bundle("Channel 1"=w40, "Channel 2"=w39, "Channel 3"=w38, "Channel 4"=w37, "Length"=w36, "SinCos"=w35, "Circle"=w34, "Pattern"=w33, "Clock counter"=w32, "SampleCount"=w31, "OptionsFieldFilter"=w30, "Output word rate"=w29) -> (w59:T16)  [unwired: 1 in]
    n233 = case shown="True" w56 {
      tunnel: w77 -> [_ w277]
      tunnel: w76 -> [_ w275]
      tunnel: w60 -> [_ w276]
      tunnel: w59 -> [_ w274]
      frame #0 {
      }
      frame #1 {
        n234 = call "SetMeasurement.vi"("int32DeviceNumber"=w275, "MeassurementSettings"=w274, "FilterSettings"=w276, "TriggerSettings"=w277) -> ("success"=w273:i32)
        n235 = Less Than 0?(x=w273) -> (x < 0?=w272:bool)
        n236 = case shown="True" w272 {
          frame #0 {
          }
          frame #1 {
            n237 = call "Meldung an Benutzer"() -> ()  [unwired: 10 in, 2 out]
          }
        }
      }
    }
    n238 = global read "Globals.vi" "boolDeviceConnected"() -> (w22:bool)
    n239 = case shown="True" "StartMeasurement" {
      frame #0 {
      }
      frame #1 {
        n240 = global read "Globals.vi" "int32DeviceNumber"() -> (w110:i32)
        n241 = call "SIOSIfmStart.vi"("deviceNumber"=w110) -> ()  [unwired: 1 out]
      }
    }
    n242 = case shown="True" "StopMeasurement" {
      frame #0 {
      }
      frame #1 {
        n243 = global read "Globals.vi" "int32DeviceNumber"() -> (w109:i32)
        n244 = call "SIOSIfmStop.vi"("deviceNumber"=w109) -> ()  [unwired: 1 out]
      }
    }
    n245 = case shown="True" w22 {
      frame #0 {
      }
      frame #1 {
        n246 = global read "Globals.vi" "int32DeviceNumber"() -> (w114:i32)
        n247 = global read "Globals.vi" "int32DeviceNumber"() -> (w120:i32)
        n248 = call "SiosIfmGetRecentValues.vi"("index"=0, "int32DeviceNumber"=w120) -> ("success"=w119:bool)
        n249 = call "SiosIfmValueCount.vi"("Device Number"=w114) -> ("Count of Values"=w113:i32)
        n250 = To Double Precision Float(number=w113) -> (double precision float=w117:dbl)
        n251 = Divide(x=w117, y=0.1) -> (x/y=→"Estimated Outputwordrate":dbl)
        n252 = Greater Than 0?(x=w113) -> (x > 0?=w118:bool)
        n253 = case shown="True" w118 {
          tunnel: w113 -> [_ w122]
          frame #0 {
          }
          frame #1 {
            n254 = for {
              N: w122 -> [_]
              n255 = global read "Globals.vi" "int32DeviceNumber"() -> (w125:i32)
              n256 = local read "Counter values"() -> (w124:bool)
              n257 = global read "Globals.vi" "SaveInFile"() -> (w123:bool)
              n258 = call "SiosIfmGetValues.vi"("Device Number"=w125) -> ()  [unwired: 1 out]
              n259 = case shown="True" w124 {
                tunnel: w123 -> [w130 w156]
                frame #0 {
                  n260 = global read "Globals.vi" "int32DeviceNumber"() -> (w131:i32)
                  n261 = call "SiosIfmLengthValue.vi"("channel"=0, "int32DeviceNumber"=w131) -> ("LengthValue"=w129:dbl)
                  n262 = call "SiosIfmLengthValue.vi"("channel"=1, "int32DeviceNumber"=w131) -> ("LengthValue"=w128:dbl)
                  n263 = call "SiosIfmLengthValue.vi"("channel"=2, "int32DeviceNumber"=w131) -> ("LengthValue"=w127:dbl)
                  n264 = call "SiosIfmLengthValue.vi"("channel"=3, "int32DeviceNumber"=w131) -> ("LengthValue"=w126:dbl)
                  n265 = case shown="True" w130 {
                    tunnel: w129 -> [_ w140]
                    tunnel: w128 -> [_ w139]
                    tunnel: w127 -> [_ w138]
                    tunnel: w126 -> [_ w137]
                    frame #0 {
                    }
                    frame #1 {
                      w144 = "\t"
                      n266 = global read "Globals.vi" "FileToSaveRefNum"() -> (w141:refnum<file>)
                      n267 = Format Value(format string="%.3f", value (0)=w140) -> (output string=w147:string)  [unwired: 1 in]
                      n268 = Format Value(format string="%.3f", value (0)=w139) -> (output string=w146:string)  [unwired: 1 in]
                      n269 = Format Value(format string="%.3f", value (0)=w138) -> (output string=w145:string)  [unwired: 1 in]
                      n270 = Format Value(format string="%.3f", value (0)=w137) -> (output string=w143:string)  [unwired: 1 in]
                      n271 = Concatenate Strings(w147, w144, w146, w144, w145, w144, w143, "\r\n") -> (w142:string)
                      n272 = Write to Text File(file (use dialog)=w141, text=w142) -> ()  [unwired: 2 in, 3 out]
                    }
                  }
                }
                frame #1 {
                  n273 = global read "Globals.vi" "int32DeviceNumber"() -> (w157:i32)
                  n274 = call "SiosIfmRawValue.vi"("channel"=0, "int32DeviceNumber"=w157) -> ("rawValue"=w155:i64)
                  n275 = call "SiosIfmRawValue.vi"("channel"=1, "int32DeviceNumber"=w157) -> ("rawValue"=w154:i64)
                  n276 = call "SiosIfmRawValue.vi"("channel"=2, "int32DeviceNumber"=w157) -> ("rawValue"=w153:i64)
                  n277 = call "SiosIfmRawValue.vi"("channel"=3, "int32DeviceNumber"=w157) -> ("rawValue"=w152:i64)
                  n278 = case shown="True" w156 {
                    tunnel: w155 -> [_ w176]
                    tunnel: w154 -> [_ w172]
                    tunnel: w153 -> [_ w171]
                    tunnel: w152 -> [_ w170]
                    frame #0 {
                    }
                    frame #1 {
                      w166 = "\t"
                      n279 = global read "Globals.vi" "FileToSaveRefNum"() -> (w163:refnum<file>)
                      n280 = Format Value(format string="%d", value (0)=w176) -> (output string=w169:string)  [unwired: 1 in]
                      n281 = Format Value(format string="%d", value (0)=w172) -> (output string=w168:string)  [unwired: 1 in]
                      n282 = Format Value(format string="%d", value (0)=w171) -> (output string=w167:string)  [unwired: 1 in]
                      n283 = Format Value(format string="%d", value (0)=w170) -> (output string=w165:string)  [unwired: 1 in]
                      n284 = Concatenate Strings(w169, w166, w168, w166, w167, w166, w165, "\r\n") -> (w164:string)
                      n285 = Write to Text File(file (use dialog)=w163, text=w164) -> ()  [unwired: 2 in, 3 out]
                    }
                  }
                }
              }
            }
          }
        }
        n286 = case shown="True" w119 {
          frame #0 {
          }
          frame #1 {
            n287 = local read "Counter values"() -> (w178:bool)
            n288 = case shown="False" w178 {
              frame #0 {
                n289 = global read "Globals.vi" "int32DeviceNumber"() -> (w182:i32)
                n290 = call "SiosIfmLengthValue.vi"("channel"=0, "int32DeviceNumber"=w182) -> ("LengthValue"=w187:dbl)
                n291 = call "SiosIfmLengthValue.vi"("channel"=1, "int32DeviceNumber"=w182) -> ("LengthValue"=w181:dbl)
                n292 = call "SiosIfmLengthValue.vi"("channel"=2, "int32DeviceNumber"=w182) -> ("LengthValue"=w180:dbl)
                n293 = call "SiosIfmLengthValue.vi"("channel"=3, "int32DeviceNumber"=w182) -> ("LengthValue"=w179:dbl)
                n294 = local write "Channel 1"(w187) -> ()
                n295 = local write "Channel 2"(w181) -> ()
                n296 = local write "Channel 3"(w180) -> ()
                n297 = local write "Channel 4"(w179) -> ()
              }
              frame #1 {
                n298 = global read "Globals.vi" "int32DeviceNumber"() -> (w191:i32)
                n299 = call "SiosIfmRawValue.vi"("channel"=0, "int32DeviceNumber"=w191) -> ("rawValue"=w195:i64)
                n300 = call "SiosIfmRawValue.vi"("channel"=1, "int32DeviceNumber"=w191) -> ("rawValue"=w190:i64)
                n301 = call "SiosIfmRawValue.vi"("channel"=2, "int32DeviceNumber"=w191) -> ("rawValue"=w189:i64)
                n302 = call "SiosIfmRawValue.vi"("channel"=3, "int32DeviceNumber"=w191) -> ("rawValue"=w188:i64)
                n303 = local write "Channel 1"(w195) -> ()
                n304 = local write "Channel 2"(w190) -> ()
                n305 = local write "Channel 3"(w189) -> ()
                n306 = local write "Channel 4"(w188) -> ()
              }
            }
          }
        }
      }
    }
    n307 = case shown="True" "SetToZero" {
      frame #0 {
      }
      frame #1 {
        n308 = global read "Globals.vi" "boolDeviceConnected"() -> (w103:bool)
        n309 = case shown="True" w103 {
          frame #0 {
          }
          frame #1 {
            n310 = global read "Globals.vi" "int32DeviceNumber"() -> (w107:i32)
            n311 = local read "Channel 1"() -> (w108:bool)
            n312 = local read "Channel 2"() -> (w106:bool)
            n313 = local read "Channel 3"() -> (w105:bool)
            n314 = local read "Channel 4"() -> (w104:bool)
            n315 = call "SiosIfmSetToZero.vi"("Channel1"=w108, "Channel2"=w106, "Channel3"=w105, "Channel4"=w104, "deviceNumber"=w107) -> ()  [unwired: 1 out]
          }
        }
      }
    }
    n316 = case shown="True" "SaveData" {
      frame #0 {
      }
      frame #1 {
        n317 = Current VI's Path() -> (path=w93:path)
        n318 = call "File Dialog"("start path"=w93, "pattern (all files)"="*.txt", "pattern label"="Textfiles") -> ("selected path"=w91:path, "cancelled"=w92:bool)  [unwired: 9 in, 2 out]
        n319 = case shown="False" w92 {
          tunnel: w91 -> [w100 _]
          frame #0 {
            n320 = Open/Create/Replace File(file path (use dialog)=w100, operation (0:open)=T9."replace or create", access (0:read/write)=enum16{"read/write", "read-only", "write-only"}."write-only") -> (refnum out=w97:refnum<file>)  [unwired: 3 in, 2 out]
            n321 = global write "Globals.vi" "FileToSaveRefNum"(w97) -> ()
            n322 = global write "Globals.vi" "SaveInFile"(TRUE ("SaveInFile")) -> ()
            n323 = property on="SaveData" class="Bool"("DisabledEnum"=T5."Disabled and Grayed Out" ("Disabled")) -> ()  [unwired: 2 in, 2 out]
            n324 = property on="StopSave" class="Bool"("DisabledEnum"=T5."Enabled" ("Disabled")) -> ()  [unwired: 2 in, 2 out]
          }
          frame #1 {
          }
        }
      }
    }
    n325 = case shown="True" "StopSave" {
      frame #0 {
      }
      frame #1 {
        n326 = global read "Globals.vi" "FileToSaveRefNum"() -> (w87:refnum<file>)
        n327 = global write "Globals.vi" "SaveInFile"(FALSE ("SaveInFile")) -> ()
        n328 = property on="SaveData" class="Bool"("DisabledEnum"=T5."Enabled" ("Disabled")) -> ()  [unwired: 2 in, 2 out]
        n329 = property on="StopSave" class="Bool"("DisabledEnum"=T5."Disabled and Grayed Out" ("Disabled")) -> ()  [unwired: 2 in, 2 out]
        n330 = Close File(refnum=w87) -> ()  [unwired: 1 in, 2 out]
      }
    }
    n331 = local read "Hardware Trigger"() -> (w52:bool)
    n332 = local read "Filter stage 1"() -> (w55:bool)
    n333 = local read "Filter stage 2"() -> (w54:bool)
    n334 = node-c288() -> ()  [unwired: 1 in, 1 out]
  }
  n335 = node-c288(w5) -> ()  [unwired: 1 out]
